vi "Ftoa, Array.vi"(5 "format (%f)":string="%f", 6 "error in":errorcluster, 8 "value":dbl[](array[numeric])) -> (0 "error out":errorcluster, 2 "string":string[](array[string]))   [LabVIEW 2010]
doc: "This function converts an Array of Doubles to an array of Strings."
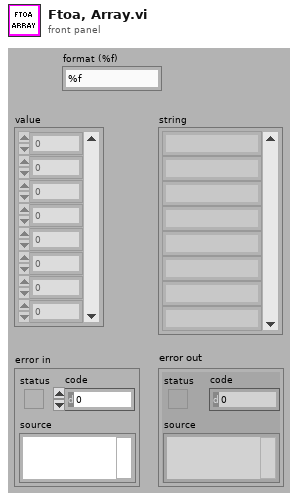
[diagram p1: front panel]
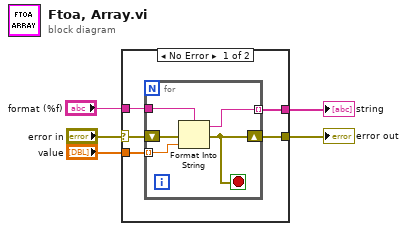
[diagram p0: block diagram]
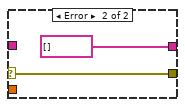
[diagram p2: hidden frame]
diagram:
  n1 = case shown="No Error" "error in" {
    selector: "error in" -> [w10 w17]
    tunnel: [w9 w17] -> w5
    tunnel: "value" -> [w8 _]
    tunnel: "format (%f)" -> [w7 _]
    tunnel: [w6 string[] []] -> w1
    frame No Error {
      n2 = for {
        shift-right: [w14] -> w9
        shift-left: w10 -> [w15]
        tunnel: w8 -> [w13] mode=indexing
        tunnel: w7 -> [w12]
        tunnel: [w11] -> w6 mode=indexing
        stop <- w14 stop-if-true
        n3 = Format Into String(format string=w12, error in=w15, w13) -> (resulting string=w11:string, error out=w14:errorcluster)  [unwired: 1 in]
      }
    }
    frame Error {
    }
  }
  "error out" <- w5
  "string" <- w1
